vi "5492_InchToEncoderPulses.vi"(8 "Encoder Clicks Per Rotation":dbl, 9 "Inches":dbl, 10 "Gear Ratio":dbl, 11 "Wheel Diameter":dbl) -> (3 "Encoder Clicks":dbl)   [LabVIEW 2016]
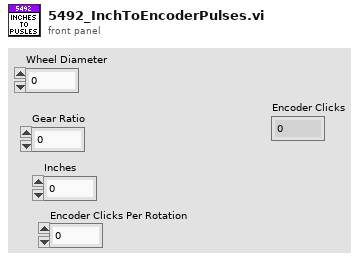
[diagram p1: front panel]
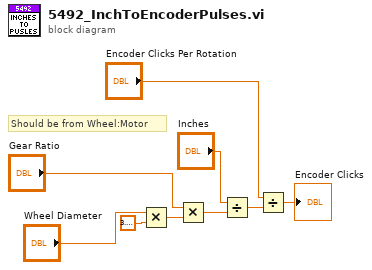
[diagram p0: block diagram]
diagram:
  # "Should be from Wheel:Motor"
  n1 = Multiply(x="Wheel Diameter", y=3.141592653589793) -> (x*y=w7:dbl)
  n2 = Multiply(x="Gear Ratio", y=w7) -> (x*y=w4:dbl)
  n3 = Divide(x="Inches", y=w4) -> (x/y=w2:dbl)
  n4 = Divide(x="Encoder Clicks Per Rotation", y=w2) -> (x/y=→"Encoder Clicks":dbl)
